vi "tsa_Predict Error Filter.vi"(8 "initial condition":dbl[](array[numeric]) format="%.2f", 9 "input signal":dbl[](array[numeric]) format="%.2f", 10 "A vector":dbl[](array[numeric]) format="%.2f", 11 "B vector":dbl[](array[numeric]) format="%.2f") -> (0 "error":i32, 3 "output signal":dbl[](array[numeric]) format="%.2f")   [LabVIEW 2020, in "NI_AALPro.lvlib"]
uses:
  NI_AALPro.lvlib
  IIR Filter with I.C. (DBL).vi
  NI_AALBase.lvlib
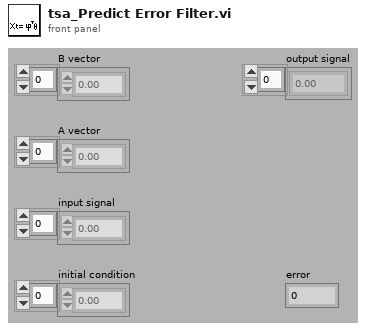
[diagram p1: front panel]
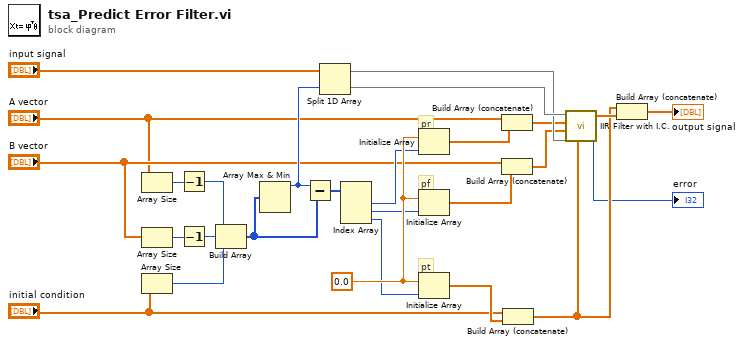
[diagram p0: block diagram]
diagram:
  w15 = 0.0
  # "pt"
  # "pf"
  # "pr"
  n1 = Array Size(array="A vector") -> (size(s)=w22:i32)
  n2 = Array Size(array="B vector") -> (size(s)=w21:i32)
  n3 = Array Size(array="initial condition") -> (size(s)=w19:i32)
  n4 = Decrement(x=w22) -> (x-1=w18:i32)
  n5 = Decrement(x=w21) -> (x-1=w20:i32)
  n6 = Build Array(w18, w20, w19) -> (w17:i32[])
  n7 = Array Max & Min(array=w17) -> (max value=w14:i32)  [unwired: 3 out]
  n8 = Subtract(x=w14, y=w17) -> (x-y=w16:i32[])
  n9 = Split 1D Array(array="input signal", index=w14) -> (first subarray=w25:dbl[], second subarray=w27:dbl[])
  n10 = Index Array(array=w16) -> (element #1=w9:i32, element #2=w8:i32, element #3=w7:i32)  [unwired: 3 in]
  n11 = Initialize Array(w15, w9) -> (w10:dbl[])
  n12 = Initialize Array(w15, w8) -> (w11:dbl[])
  n13 = Initialize Array(w15, w7) -> (w12:dbl[])
  n14 = Build Array (concatenate)("A vector", w10) -> (w24:dbl[])
  n15 = Build Array (concatenate)("B vector", w11) -> (w23:dbl[])
  n16 = Build Array (concatenate)("initial condition", w12) -> (w13:dbl[])
  n17 = call-poly "IIR Filter with I.C..vi"("Initial Y Conditions"=w13, "Initial X Conditions"=w25, "Forward Coefficients"=w23, "Reverse Coefficients"=w24, "X"=w27) -> ("error"=→"error":i32, "Filtered X"=w26:dbl[])  [unwired: 2 in, 2 out]
  n18 = Build Array (concatenate)(w13, w26) -> (→"output signal":dbl[])
